vi "SetPosition.vi"(7 "Index":i16, 8 "error in (no error)":errorcluster, 9 "Y":i16, 10 "X":i16, 11 "SpriteHandler in":refnum<class "SpriteHandler.lvclass">) -> (0 "error out":errorcluster, 3 "SpriteHandler out":refnum<class "SpriteHandler.lvclass">)   [LabVIEW 2019, in "RT_Game.lvlib" / "SpriteHandler.lvclass"]
uses:
  SpriteHandler.lvclass
  SpriteHandler.lvclass/SpriteHandler.ctl
  RT_Sprite/RT_Sprite.lvclass
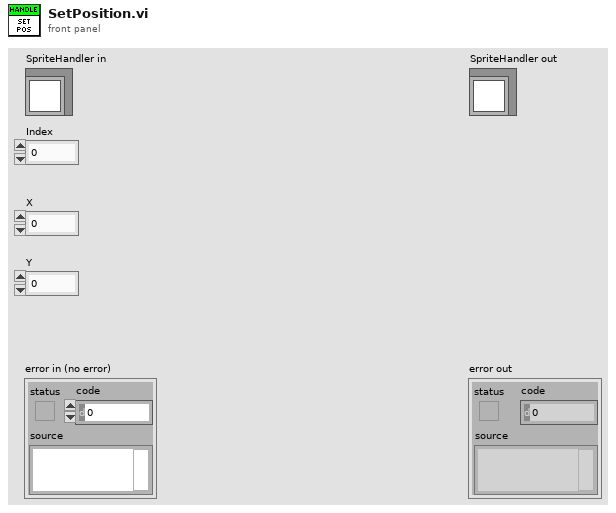
[diagram p1: front panel]
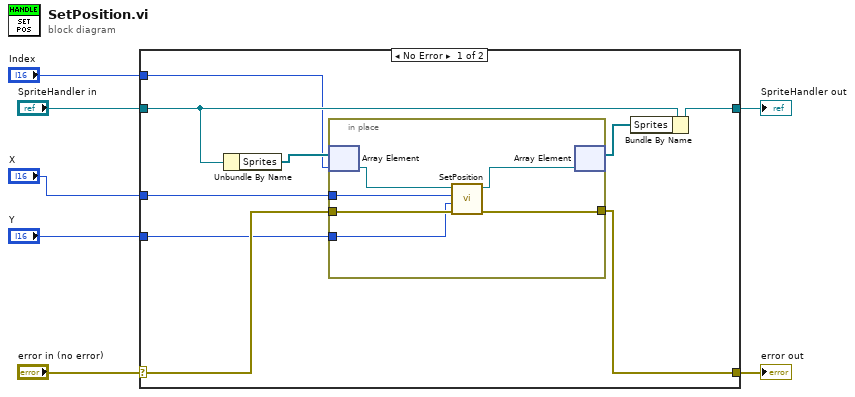
[diagram p0: block diagram]
diagram:
  n1 = case shown="No Error" "error in (no error)" {
    selector: "error in (no error)" -> [w11 w24]
    tunnel: [w10 w24] -> w6
    tunnel: [w13 w23] -> w4
    tunnel: "SpriteHandler in" -> [w16 w23]
    tunnel: "Index" -> [w14 _]
    tunnel: "X" -> [w9 _]
    tunnel: "Y" -> [w8 _]
    frame No Error {
      n2 = Unbundle By Name(w16) -> ("Sprites"=w15:refnum<class "RT_Sprite.lvclass">[])
      n3 = in-place {
        in-place-border: w11 -> [w22]
        in-place-border: [w21] -> w10
        in-place-border: w9 -> [w18]
        in-place-border: w8 -> [w17]
        n4 = in-place-array #1(w15, w14) -> (w20:refnum<class "RT_Sprite.lvclass">)
        n5 = call "SetPosition.vi"("error in (no error)"=w22, "Y"=w17, "X"=w18, "RT_Sprite in"=w20) -> ("error out"=w21:errorcluster, "RT_Sprite out"=w19:refnum<class "RT_Sprite.lvclass">)  [unwired: 6 in]
        n6 = in-place-array #1(w19) -> (w12:refnum<class "RT_Sprite.lvclass">[])  [unwired: 1 out]
      }
      n7 = Bundle By Name(cluster=w16, "Sprites"=w12) -> (w13:refnum<class "SpriteHandler.lvclass">)
    }
    frame Error {
    }
  }
  "error out" <- w6
  "SpriteHandler out" <- w4
